vi "calculator.vi"() -> ()   [LabVIEW 2012]
panel:
  in  "Enum SIGN to case":enum16{"+", "-", "X", "/"}(ring)
  out "RESULT":dbl
  in  "NUMBER 2":dbl
  in  "NUMBER 1":dbl
  in  "stop":bool
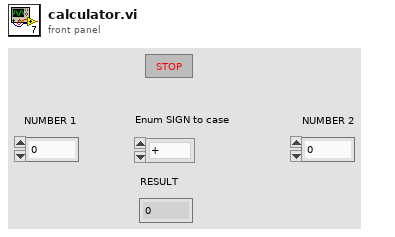
[diagram p1: front panel]
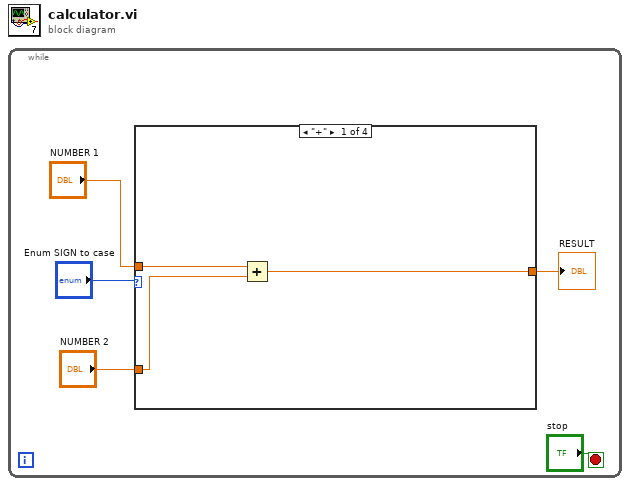
[diagram p0: block diagram]
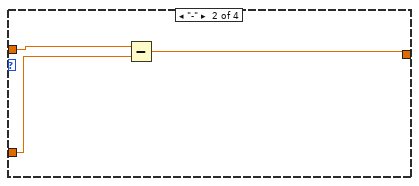
[diagram p2: hidden frame]
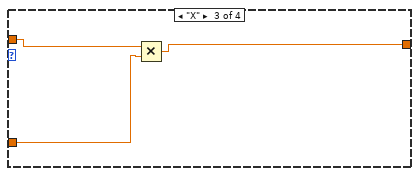
[diagram p3: hidden frame]
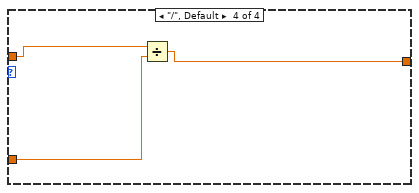
[diagram p4: hidden frame]
diagram:
  n1 = while {
    stop <- "stop" stop-if-true
    n2 = case shown="\"+\"" "Enum SIGN to case" {
      tunnel: "NUMBER 1" -> [w8 w11 w14 w17]
      tunnel: "NUMBER 2" -> [w7 w10 w13 w16]
      tunnel: [w6 w9 w12 w15] -> w2
      frame "+" {
        n3 = Add(x=w8, y=w7) -> (x+y=w6:dbl)
      }
      frame "-" {
        n4 = Subtract(x=w11, y=w10) -> (x-y=w9:dbl)
      }
      frame "X" {
        n5 = Multiply(x=w14, y=w13) -> (x*y=w12:dbl)
      }
      frame "/", Default {
        n6 = Divide(x=w17, y=w16) -> (x/y=w15:dbl)
      }
    }
    "RESULT" <- w2
  }
